vi "参数设置页.vi"() -> ()   [LabVIEW 2016, in "斯坦道总磷.lvlib"]
uses:
  <vilib>/Plasmionique/MB Master/MB_Master/MB_Master.lvclass
  <vilib>/ptbypt/NI_PtbyPt.lvlib
panel:
  in  "简易流程路径":path=path "data/流程.xml"
  out "数据刷新时间":string
  in  "通讯连接":bool
  out "MB table":enum32{"Serial", "TCP"}(tab)
  in  "请选择串口:":refnum<visa-resource-name>
  in  "IP":string="127.0.0.1"
  in  "PORT":string="1001"
  in  "通信方式选择":enum16{"串口", "TCP"}(ring)
  in  "盐度自动补偿：":bool
  out "盐度补偿值":dbl caption="盐度补偿值："
  in  "刷新":bool
  in  "测量模式":T1(ring)
  in  "参数下拉列表":u16(ring)
  in  "量程下拉列表":enum16{"低量程", "高量程"}(ring)
  in  "测试流程路径":path=path "data/流程.xml"
  in  "标样核查量程模式":enum16{"高量程", "低量程", "自动"}(ring) caption="标样核查量程模式："
  in  "加标回收量程模式":enum16{"高量程", "低量程", "自动"}(ring) caption="加标回收量程模式："
  in  "跨度核查量程模式":enum16{"高量程", "低量程", "自动"}(ring) caption="跨度核查量程模式："
  in  "零点核查量程模式":enum16{"高量程", "低量程", "自动"}(ring) caption="零点核查量程模式："
  in  "水样测试量程模式":enum16{"高量程", "低量程", "自动"}(ring) caption="水样测试量程模式："
  out "稀释度":dbl caption="稀释度："
  out "阈值（高->低）":dbl caption="阈值（高->低）："
  out "阈值（低->高）":dbl caption="阈值（低->高）："
  out "量程下限":dbl caption="量程下限："
  out "量程上限":dbl caption="量程上限："
  out "检出限":dbl caption="检出限："
  out "曲线截距":dbl caption="曲线截距：" format="%#.6f"
  out "曲线斜率":dbl caption="曲线斜率：" format="%#.6f"
  out "二次多项式系数":dbl caption="二次多项式系数：" format="%#.6f"
  out "消解时长":dbl caption="消解时长："
  out "消解温度":dbl caption="消解温度："
  out "测量精度":u16 caption="测量精度："
  in  "标样核查标液浓度":dbl caption="标样核查标液浓度："
  in  "跨度核查标液浓度":dbl caption="跨度核查标液浓度："
  in  "零点核查标液浓度":dbl caption="零点核查标液浓度："
  in  "跨度值":dbl caption="跨度值："
  # "ppt"
  # "mg/L"
  # "mg/L"
  # "mg/L"
  # "mg/L"
  # "mg/L"
  # "min"
  # "℃"
  # "mg/L"
  # "mg/L"
  # "mg/L"
  # "mg/L"
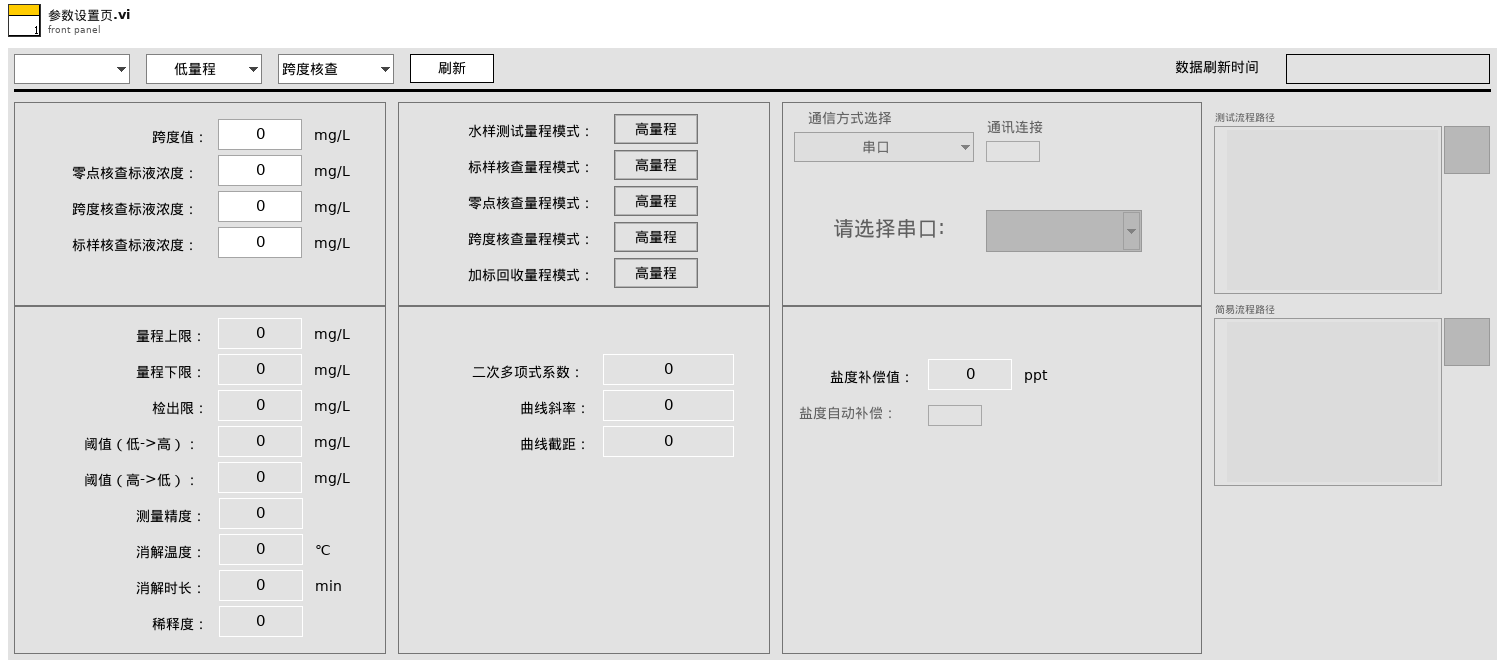
[diagram p1: front panel]
types:
  T1 = enum16{"跨度核查", "水样测量", "零点核查", "标样核查", "加标回收", "快捷测试", "空白校准", "标样校准"}
  T2 = typedef "LVStringsAndValuesArrayTypeDef_U16.ctl" = cluster{"String":string, "Value":u16}[]
  T3 = cluster{"系统时间":timestamp, "工作状态":u16, "测量模式":enum16{"待机", "连续模式", "周期模式", "定点模式", "受控模式", "手动模式"}, "告警代码":u16, "故障代码":u16, "日志代码":u16, "软件版本":u16, "F0":sgl, "F1":sgl, "F2":sgl, "F3":sgl, "T":sgl, "H":sgl, "id":u16, "flowid":u16, "量程":u16, "总磷控温温度1":sgl, "营养盐控温温度2":sgl, "ADC":sgl}
  T4 = enum8{"Enabled", "Disabled", "Disabled and Grayed Out"}
  T5 = cluster{"测量精度":u16, "检出限":dbl, "上限":dbl, "下限":dbl, "阈值（低->高）":dbl, "阈值（高->低）":dbl, "稀释度":dbl}
  T6 = cluster{"泵类型":u8, "进样速度":u32, "出样速度":u32, "泵阀量":u8, "光谱仪类型":u8, "光谱采样次数":u8, "氙灯次数":u8, "B":u16, "C":u16, "D":u16, "E":u16, "B_COD":u16, "C_COD":u16, "D_COD":u16, "E_COD":u16, "G":u16, "M":u16, "N":u16, "氨氮注射泵控温下限":sgl, "氨氮注射泵控温上限":sgl, "总氮注射泵控温下限":sgl, "总氮注射泵控温上限":sgl, "消解温度下限":sgl, "消解温度上限":sgl, "加热10s限值":sgl, "高温高压阀开阀温度":sgl, "总氮x公式0":u8, "总氮x公式1":sgl, "总氮x公式2":sgl, "总磷浊度稀释系数":sgl, "总磷浊度补偿权重1":sgl, "总磷浊度补偿权重2":sgl, "盐度系数":sgl, "氨氮补偿系数1":sgl, "氨氮补偿系数2":sgl}
  T7 = cluster{"水样测试量程模式":enum16{"高量程", "低量程", "自动"}, "零点核查量程模式":enum16{"高量程", "低量程", "自动"}, "跨度核查量程模式":enum16{"高量程", "低量程", "自动"}, "加标回收量程模式":enum16{"高量程", "低量程", "自动"}, "标样核查量程模式":enum16{"高量程", "低量程", "自动"}}
  T8 = cluster{"水样测试量程模式":u16, "零点核查量程模式":u16, "跨度核查量程模式":u16, "加标回收量程模式":u16, "标样核查量程模式":u16}
  T9 = cluster{"总磷跨度值":dbl, "总磷零点标准液浓度":dbl, "总磷跨度标准液浓度":dbl, "总磷标准液标准浓度":dbl, "总氮跨度值":dbl, "总氮零点标准液浓度":dbl, "总氮跨度标准液浓度":dbl, "总氮标准液标准浓度":dbl, "COD跨度值":dbl, "COD零点标准液浓度":dbl, "COD跨度标准液浓度":dbl, "COD标准液标准浓度":dbl, "氨氮跨度值":dbl, "氨氮零点标准液浓度":dbl, "氨氮跨度标准液浓度":dbl, "氨氮标准液标准浓度":dbl, "磷酸盐跨度值":dbl, "磷酸盐零点标准液浓度":dbl, "磷酸盐跨度标准液浓度":dbl, "磷酸盐标准液标准浓度":dbl, "硝氮跨度值":dbl, "硝氮零点标准液浓度":dbl, "硝氮跨度标准液浓度":dbl, "硝氮标准液标准浓度":dbl, "亚硝氮跨度值":dbl, "亚硝氮零点标准液浓度":dbl, "亚硝氮跨度标准液浓度":dbl, "亚硝氮标准液标准浓度":dbl, "硫化物跨度值":dbl, "硫化物零点标准液浓度":dbl, "硫化物跨度标准液浓度":dbl, "硫化物标准液标准浓度":dbl, "硅酸盐跨度值":dbl, "硅酸盐零点标准液浓度":dbl, "硅酸盐跨度标准液浓度":dbl, "硅酸盐标准液标准浓度":dbl}
  T10 = cluster{"水样测试量程模式":enum16{"H", "L", "AUTO"}, "空白核查量程模式":enum16{"H", "L", "AUTO"}, "跨度核查量程模式":enum16{"H", "L", "AUTO"}, "加标回收量程模式":enum16{"H", "L", "AUTO"}, "标样核查量程模式":enum16{"H", "L", "AUTO"}}
  T11 = cluster{"水样测试量程模式":u16, "空白核查量程模式":u16, "跨度核查量程模式":u16, "加标回收量程模式":u16, "标样核查量程模式":u16}
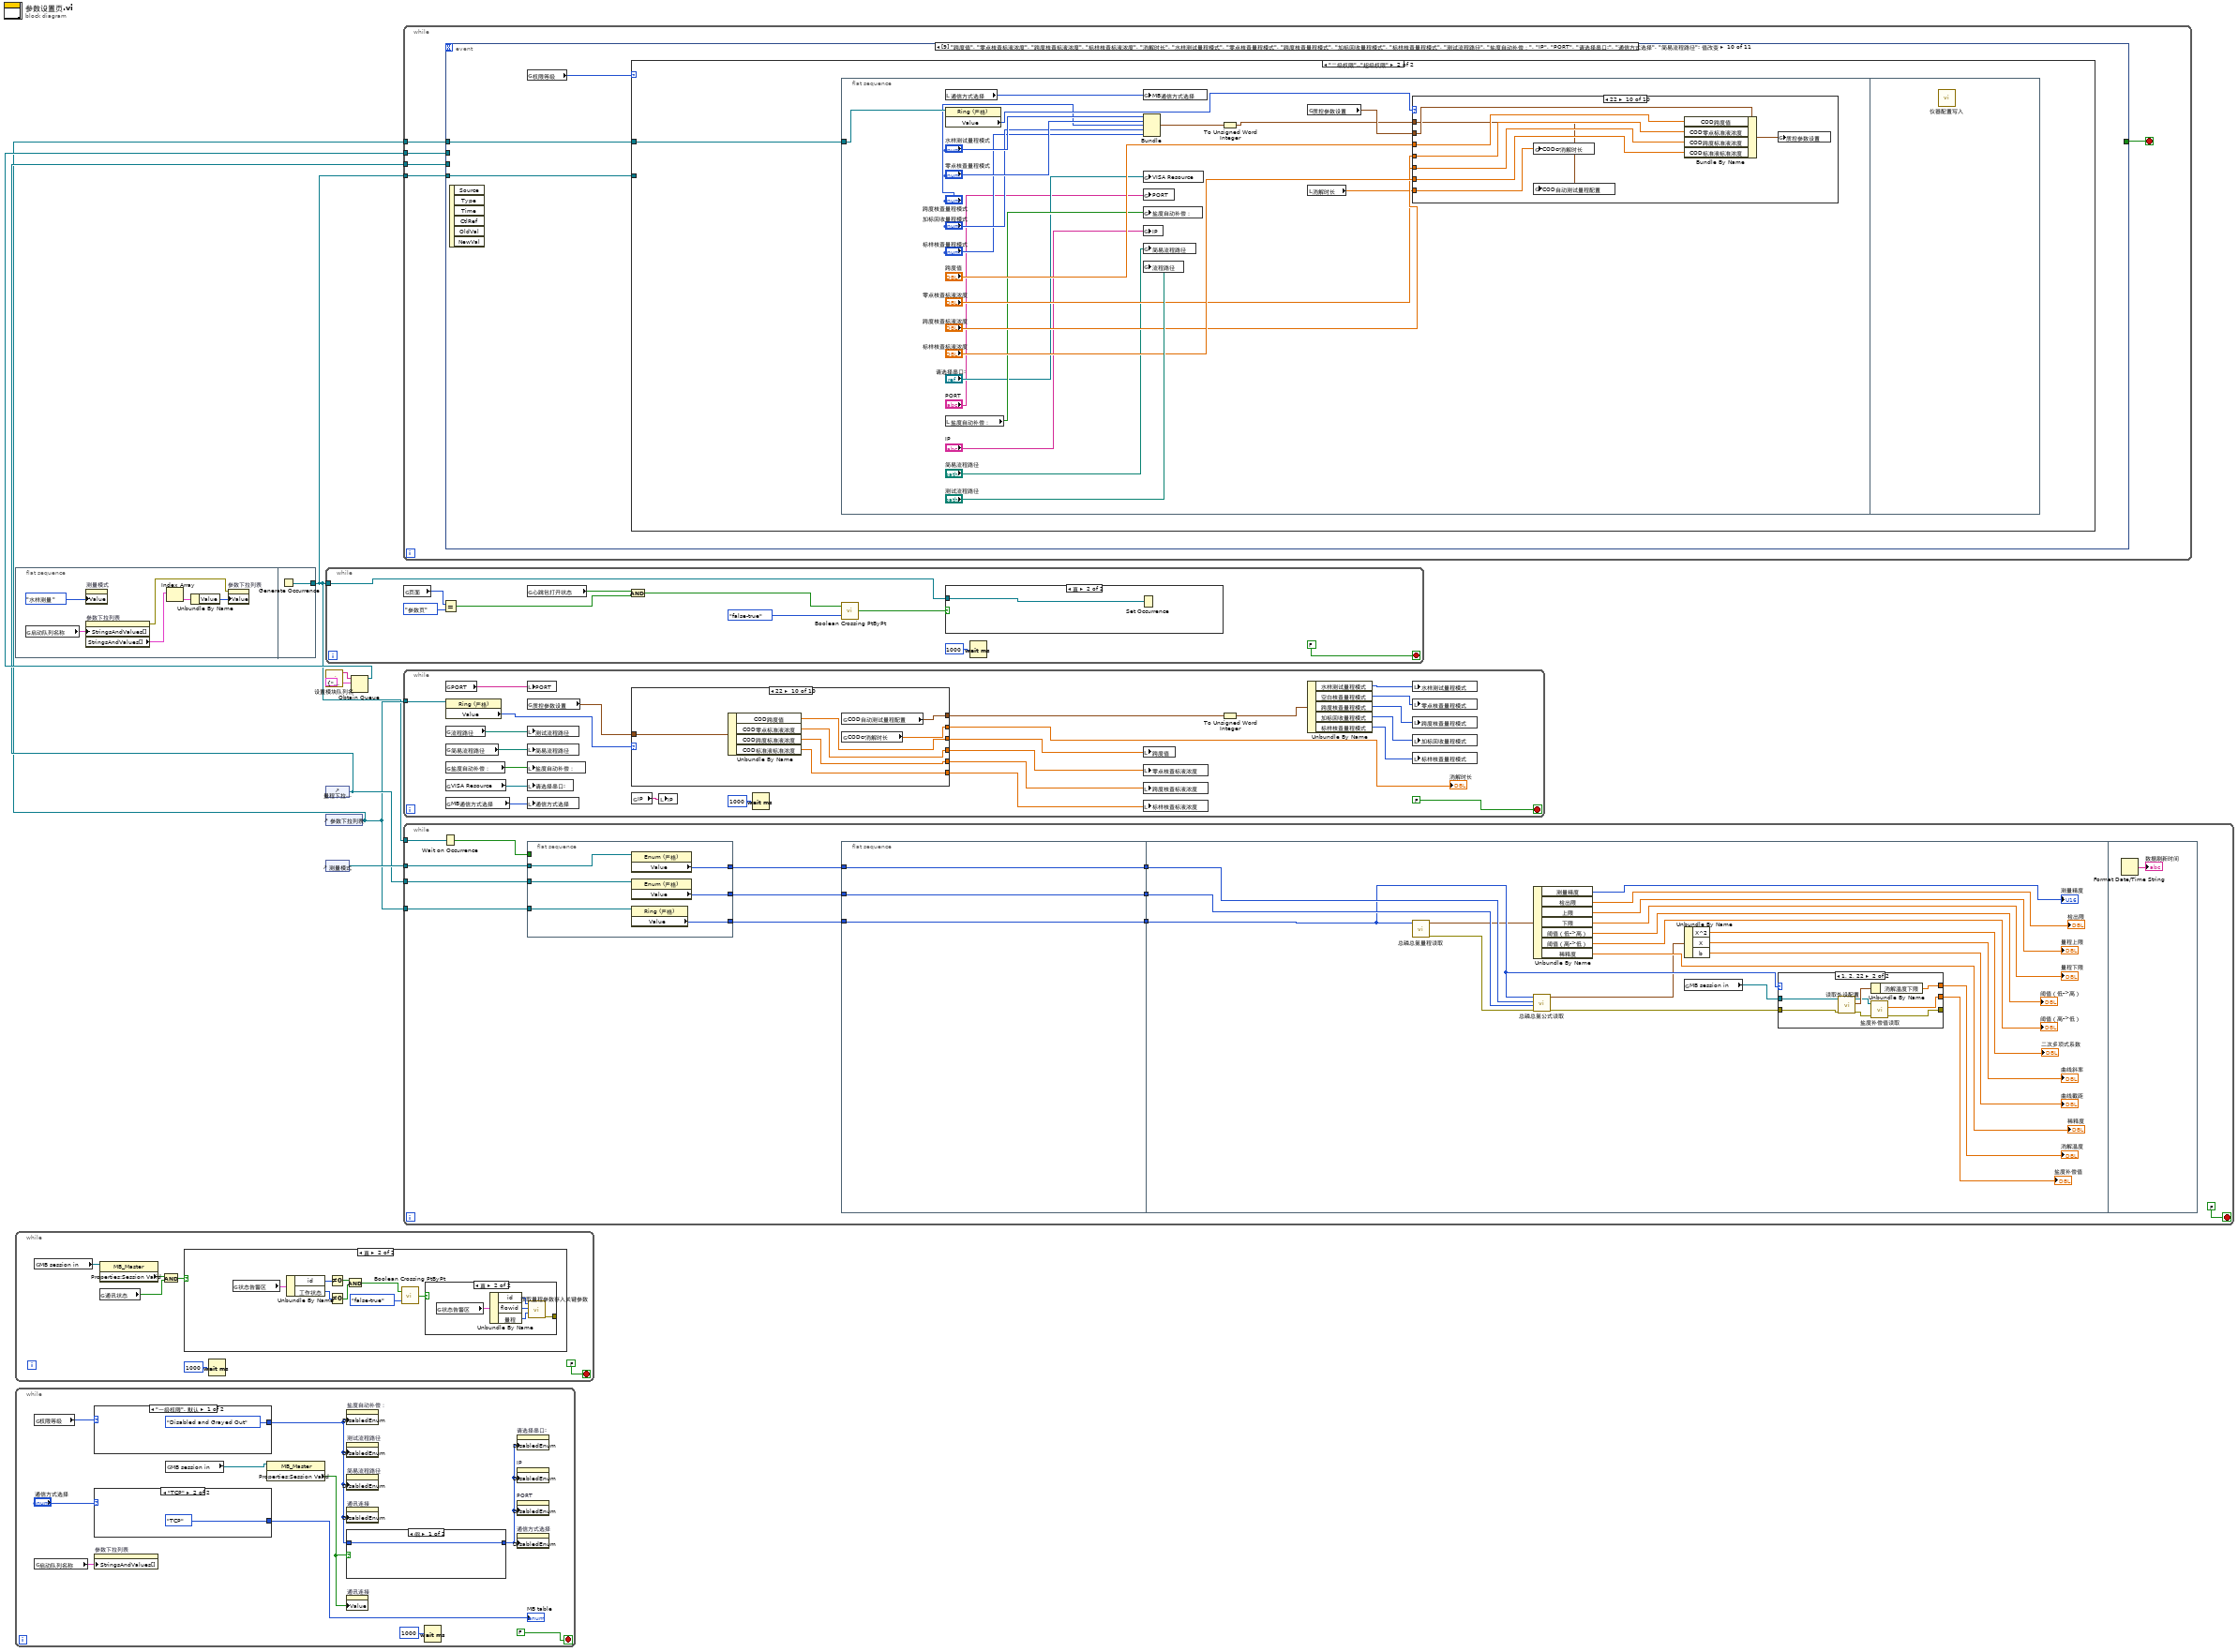
[diagram p0: block diagram]
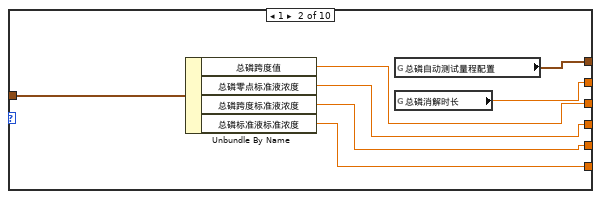
[diagram p6: hidden frame]
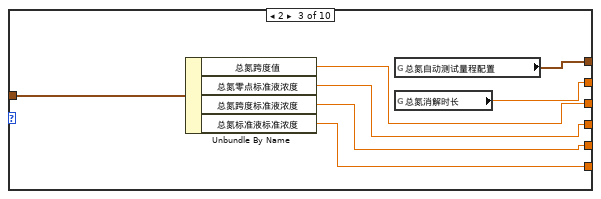
[diagram p7: hidden frame]
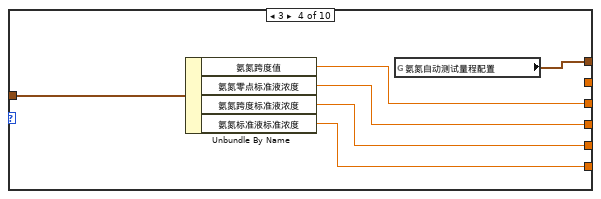
[diagram p8: hidden frame]
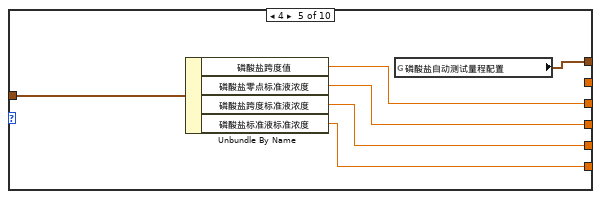
[diagram p9: hidden frame]
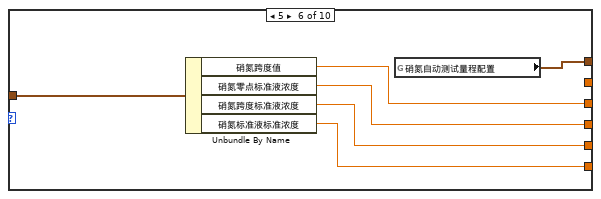
[diagram p10: hidden frame]
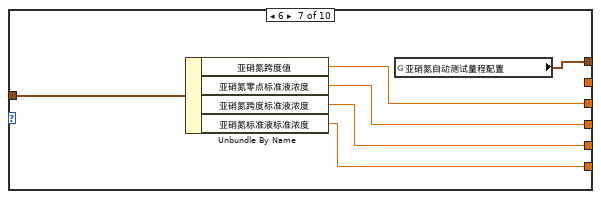
[diagram p11: hidden frame]
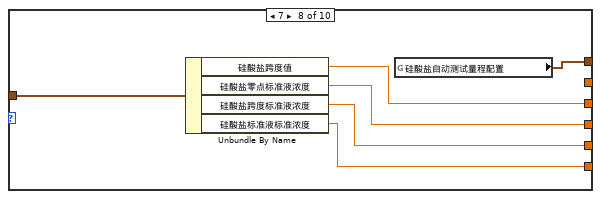
[diagram p12: hidden frame]
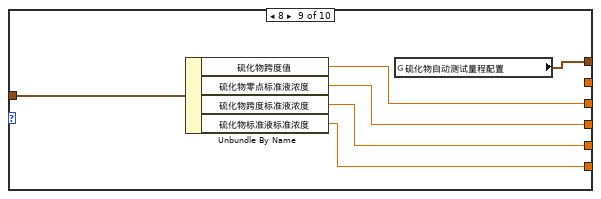
[diagram p13: hidden frame]
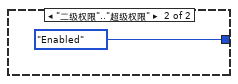
[diagram p14: hidden frame]
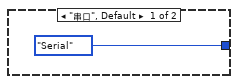
[diagram p15: hidden frame]
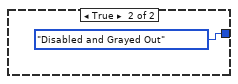
[diagram p16: hidden frame]
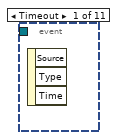
[diagram p17: hidden frame]
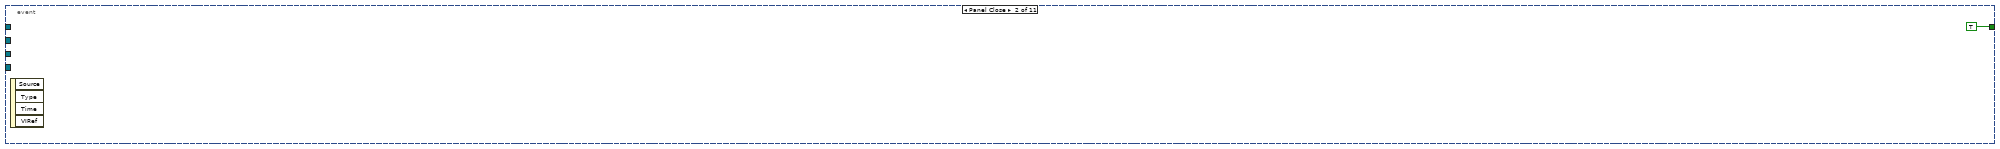
[diagram p18: hidden frame]
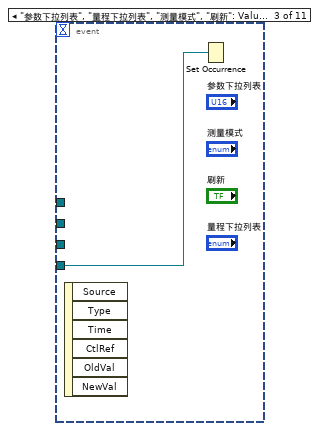
[diagram p19: hidden frame]
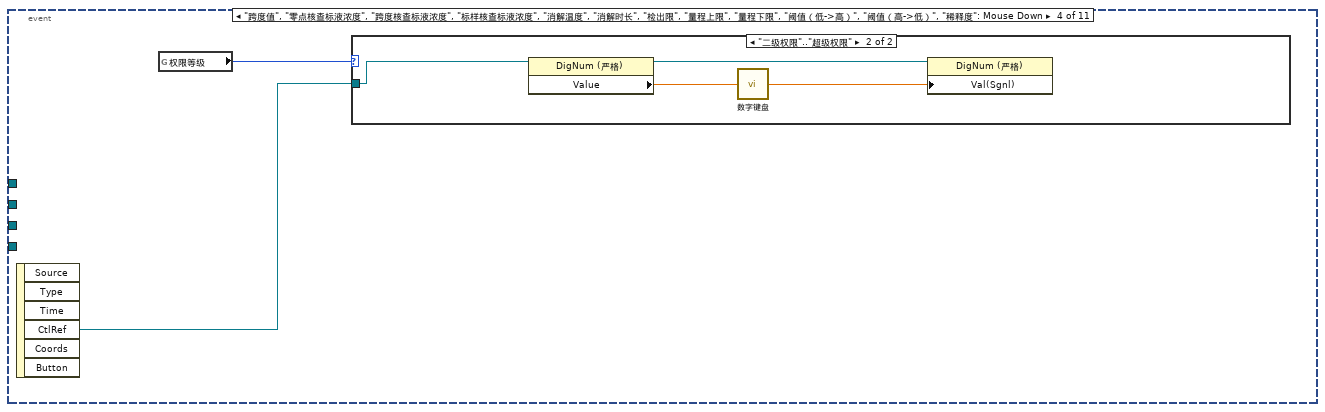
[diagram p20: hidden frame]
diagram:
  n1 = flat-sequence {
    tunnel: [w14] -> w1
    frame #0 {
      n2 = global read "model config var.vi" "启动队列名称"() -> (w9:cluster{"String":string, "Value":u16}[])
      n3 = property on="测量模式" class="Enum (严格)"("Value"=T1."水样测量" ("测量模式")) -> ()  [unwired: 2 in, 2 out]
      n4 = property on="参数下拉列表" class="Ring (严格)"("StringsAndValues[]"=w9) -> (error out=w12:errorcluster, "StringsAndValues[]"=w10:T2)  [unwired: 2 in, 1 out]
      n5 = Index Array(array=w10) -> (element=w11:cluster{"String":string, "Value":u16})  [unwired: 1 in]
      n6 = Unbundle By Name(w11) -> ("Value"=w13:u16)
      n7 = property on="参数下拉列表" class="Ring (严格)"(error in=w12, "Value"=w13) -> ()  [unwired: 1 in, 2 out]
    }
    frame #1 {
      n8 = Generate Occurrence() -> (w14:refnum<k4>)
    }
  }
  n9 = while {
    stop <- FALSE stop-if-true
    n10 = global read "VAR总磷总氮全局变量.vi" "MB session in"() -> (w17:refnum<class "MB_Master.lvclass">)
    n11 = property class="MB_Master"(reference=w17) -> ("Properties:Session Valid"=w15:bool)  [unwired: 1 in, 2 out]
    n12 = global read "VAR总磷总氮全局变量.vi" "通讯状态"() -> (w19:bool)
    n13 = And(x=w15, y=w19) -> (x .and. y?=w16:bool)
    n14 = case shown="真" w16 {
      frame False {
      }
      frame True {
        n15 = global read "VAR总磷总氮全局变量.vi" "状态告警区"() -> (w28:T3)
        n16 = Unbundle By Name(w28) -> ("id"=w22:u16, "工作状态"=w27:u16)
        n17 = Not Equal To 0?(x=w22) -> (x != 0?=w23:bool)
        n18 = Not Equal To 0?(x=w27) -> (x != 0?=w24:bool)
        n19 = And(x=w23, y=w24) -> (x .and. y?=w25:bool)
        n20 = call <vilib>:"Boolean Crossing PtByPt.vi"("direction"=enum16{"either", "false-true", "true-false"}."false-true", "input"=w25) -> ("crossing"=w21:bool)  [unwired: 1 in]
        n21 = case shown="真" w21 {
          tunnel: [_ w33] -> _
          frame False {
          }
          frame True {
            n22 = global read "VAR总磷总氮全局变量.vi" "状态告警区"() -> (w32:T3)
            n23 = Unbundle By Name(w32) -> ("id"=w31:u16, "flowid"=w30:u16, "量程"=w29:u16)
            n24 = call "获取量程参数存入关键参数.vi"("量程"=w29, "flowid"=w30, "id"=w31) -> ("error out"=w33:errorcluster)  [unwired: 8 in]
          }
        }
      }
    }
    n25 = Wait (ms)(milliseconds to wait=u32 1000 ("等待时间（毫秒）")) -> ()  [unwired: 1 out]
  }
  n26 = while {
    stop <- FALSE stop-if-true
    n27 = global read "VAR总磷总氮全局变量.vi" "权限等级"() -> (w36:enum16{"一级权限", "二级权限", "三级权限", "超级权限"})
    n28 = global read "model config var.vi" "启动队列名称"() -> (w34:cluster{"String":string, "Value":u16}[])
    n29 = case shown="\"一级权限\", 默认" w36 {
      tunnel: [T4."Disabled and Grayed Out" ("禁用") T4."Enabled" ("禁用")] -> w35
      frame "一级权限", Default {
      }
      frame "二级权限".."超级权限" {
      }
    }
    n30 = case shown="\"TCP\"" "通信方式选择" {
      tunnel: [enum32{"Serial", "TCP"}."Serial" ("MB table") enum32{"Serial", "TCP"}."TCP" ("MB table")] -> w38
      frame "串口", Default {
      }
      frame "TCP" {
      }
    }
    "MB table" <- w38
    n31 = property on="参数下拉列表" class="Ring (严格)"("StringsAndValues[]"=w34) -> ()  [unwired: 2 in, 2 out]
    n32 = global read "VAR总磷总氮全局变量.vi" "MB session in"() -> (w42:refnum<class "MB_Master.lvclass">)
    n33 = property class="MB_Master"(reference=w42) -> ("Properties:Session Valid"=w40:bool)  [unwired: 1 in, 2 out]
    n34 = property on="盐度自动补偿：" class="Bool (严格)"("DisabledEnum"=w35) -> ()  [unwired: 2 in, 2 out]
    n35 = property on="测试流程路径" class="Path"("DisabledEnum"=w35) -> ()  [unwired: 2 in, 2 out]
    n36 = property on="简易流程路径" class="Path"("DisabledEnum"=w35) -> ()  [unwired: 2 in, 2 out]
    n37 = property on="通讯连接" class="Bool (严格)"("DisabledEnum"=w35) -> ()  [unwired: 2 in, 2 out]
    n38 = case shown="假" w40 {
      tunnel: [w48 T4."Disabled and Grayed Out" ("禁用")] -> w39
      tunnel: w35 -> [w48 _]
      frame False {
      }
      frame True {
      }
    }
    n39 = property on="通讯连接" class="Bool (严格)"("Value"=w40) -> ()  [unwired: 2 in, 2 out]
    n40 = Wait (ms)(milliseconds to wait=u32 1000 ("等待时间（毫秒）")) -> ()  [unwired: 1 out]
    n41 = property on="请选择串口:" class="VISAName"("DisabledEnum"=w39) -> ()  [unwired: 2 in, 2 out]
    n42 = property on="IP" class="Str"("DisabledEnum"=w39) -> ()  [unwired: 2 in, 2 out]
    n43 = property on="PORT" class="Str"("DisabledEnum"=w39) -> ()  [unwired: 2 in, 2 out]
    n44 = property on="通信方式选择" class="Enum (严格)"("DisabledEnum"=w39) -> ()  [unwired: 2 in, 2 out]
  }
  n45 = while {
    tunnel: w1 -> [w56]
    stop <- FALSE stop-if-true
    n46 = global read "VAR总磷总氮全局变量.vi" "页面"() -> (w58:enum16{"主页", "参数页", "校准页"})
    n47 = Equal?(x=w58, y=enum16{"主页", "参数页", "校准页"}."参数页" ("页面")) -> (x = y?=w57:bool)
    n48 = global read "VAR总磷总氮全局变量.vi" "心跳包打开状态"() -> (w52:bool)
    n49 = And(x=w52, y=w57) -> (x .and. y?=w53:bool)
    n50 = call <vilib>:"Boolean Crossing PtByPt.vi"("direction"=enum16{"either", "false-true", "true-false"}."false-true", "input"=w53) -> ("crossing"=w51:bool)  [unwired: 1 in]
    n51 = case shown="真" w51 {
      tunnel: w56 -> [_ w60]
      frame False {
      }
      frame True {
        n52 = Set Occurrence(w60) -> ()
      }
    }
    n53 = Wait (ms)(milliseconds to wait=u32 1000 ("等待时间（毫秒）")) -> ()  [unwired: 1 out]
  }
  n54 = call "设置模块队列名.vi"() -> ("Msg"=w6:string)  [unwired: 5 in]
  n55 = control-ref of="量程下拉列表"() -> (w3:refnum<vi>)
  n56 = control-ref of="参数下拉列表"() -> (w2:refnum<vi>)
  n57 = control-ref of="测量模式"() -> (w4:refnum<vi>)
  n58 = Obtain Queue(name (unnamed)=w6, element data type=cluster{"命令":string, "data":variant} {"命令"="", "data"=variant}) -> (queue out=w5:refnum<queue>)  [unwired: 3 in, 2 out]
  n59 = while {
    tunnel: w1 -> [w64]
    tunnel: w2 -> [w63]
    tunnel: w5 -> [w62]
    tunnel: w3 -> [w61]
    stop <- w65 stop-if-true
    n60 = event shown="[9] \"跨度值\", \"零点核查标液浓度\", \"跨度核查标液浓度\", \"标样核查标液浓度\", \"消解时长\", \"水样测试量程模式\", \"零点核查量程模式\", \"跨度核查量程模式\", \"加标回收量程模式\", \"标样核查量程模式\", \"测试流程路径\", \"盐度自动补偿：\", \"IP\", \"PORT\", \"请选择串口:\", \"通信方式选择\", \"简易流程路径\": 值改变" {
      selector: _ -> [_ _ _ _ _ _ _ _ _ _ _]
      dyn-events: _ -> [_ _ _ _ _ _ _ _ _ _ _]
      timeout: _ -> [_ _ _ _ _ _ _ _ _ _ _]
      tunnel: [_ TRUE _ _ _ _ _ _ _ _ _] -> w65
      tunnel: w64 -> [_ _ w67 _ _ _ _ _ _ w114 _]
      tunnel: w63 -> [_ _ _ _ w86 _ _ _ _ w116 _]
      tunnel: w62 -> [_ _ _ _ _ _ _ _ _ _ w208]
      tunnel: w61 -> [_ _ _ _ _ _ _ _ _ _ _]
      event Timeout {
        n61 = event-data() -> ()  [unwired: 1 in, 3 out]
      }
      event Panel Close {
        n62 = event-data() -> ()  [unwired: 1 in, 4 out]
      }
      event "参数下拉列表", "量程下拉列表", "测量模式", "刷新": Value Change {
        n63 = event-data() -> ()  [unwired: 1 in, 6 out]
        n64 = Set Occurrence(w67) -> ()
      }
      event "跨度值", "零点核查标液浓度", "跨度核查标液浓度", "标样核查标液浓度", "消解温度", "消解时长", "检出限", "量程上限", "量程下限", "阈值（低->高）", "阈值（高->低）", "稀释度": Mouse Down {
        n65 = event-data() -> ("CtlRef"=w69:refnum<vi>)  [unwired: 1 in, 5 out]
        n66 = global read "VAR总磷总氮全局变量.vi" "权限等级"() -> (w68:enum16{"一级权限", "二级权限", "三级权限", "超级权限"})
        n67 = case shown="\"二级权限\"..\"超级权限\"" w68 {
          tunnel: w69 -> [_ w73]
          frame "一级权限", Default {
          }
          frame "二级权限".."超级权限" {
            n68 = property class="DigNum (严格)"(reference=w73) -> (reference out=w71:refnum<vi>, "Value"=w72:dbl)  [unwired: 1 in, 1 out]
            n69 = call "数字键盘.vi"("OldNumber"=w72) -> ("NewNumber"=w70:dbl)
            n70 = property class="DigNum (严格)"(reference=w71, "Val(Sgnl)"=w70) -> ()  [unwired: 1 in, 2 out]
          }
        }
      }
      event "测量精度", "检出限", "量程上限", "量程下限", "阈值（低->高）", "阈值（高->低）", "稀释度": Value Change {
        n71 = event-data() -> ()  [unwired: 1 in, 6 out]
        n72 = local read "测量精度"() -> (w76:u16)
        n73 = local read "检出限"() -> (w80:dbl)
        n74 = local read "量程上限"() -> (w82:dbl)
        n75 = local read "量程下限"() -> (w81:dbl)
        n76 = local read "阈值（低->高）"() -> (w79:dbl)
        n77 = local read "阈值（高->低）"() -> (w78:dbl)
        n78 = local read "稀释度"() -> (w77:dbl)
        n79 = property class="Ring (严格)"(reference=w86) -> ("Value"=w85:u16)  [unwired: 1 in, 2 out]
        n80 = Bundle By Name(cluster=T5 {"测量精度"=0, "检出限"=0.0, "上限"=0.0, "下限"=0.0, "阈值（低->高）"=0.0, "阈值（高->低）"=0.0, "稀释度"=0.0} ("量程参数写入"), "测量精度"=w76, "检出限"=w80, "上限"=w82, "下限"=w81, "阈值（低->高）"=w79, "阈值（高->低）"=w78, "稀释度"=w77) -> (w83:T5)
        n81 = call "总磷总氮量程写入.vi"("量程参数写入"=w83, "测量参数"=w85) -> ("error out"=w74:errorcluster)  [unwired: 8 in]
        n82 = case shown="错误" w74 {
          tunnel: ["写入成功" "写入失败"] -> w75
          frame No Error {
          }
          frame Error {
          }
        }
        n83 = One Button Dialog(message=w75) -> ()  [unwired: 1 in, 1 out]
      }
      event "消解温度": Value Change {
        n84 = event-data() -> ("NewVal"=w91:dbl)  [unwired: 1 in, 5 out]
        n85 = global read "VAR总磷总氮全局变量.vi" "MB session in"() -> (w92:refnum<class "MB_Master.lvclass">)
        n86 = call "读取外设配置.vi"("MB session in"=w92) -> ("error out"=w95:errorcluster, "外设配置"=w94:T6)  [unwired: 8 in, 1 out]
        n87 = Bundle By Name(cluster=w94, "消解温度下限"=w91) -> (w93:T6)
        n88 = call "写入外设配置.vi"("error in (no error)"=w95, "外设配置"=w93, "MB session in"=w92) -> ("error out"=w90:errorcluster)  [unwired: 7 in, 1 out]
        n89 = case shown="错误" w90 {
          tunnel: ["写入成功" "写入失败"] -> w89
          frame No Error {
          }
          frame Error {
          }
        }
        n90 = One Button Dialog(message=w89) -> ()  [unwired: 1 in, 1 out]
      }
      event "测量精度": Mouse Down {
        n91 = event-data() -> ("CtlRef"=w99:refnum<vi>)  [unwired: 1 in, 7 out]
        n92 = global read "VAR总磷总氮全局变量.vi" "权限等级"() -> (w98:enum16{"一级权限", "二级权限", "三级权限", "超级权限"})
        n93 = case shown="\"二级权限\"..\"超级权限\"" w98 {
          tunnel: w99 -> [_ w103]
          frame "一级权限", Default {
          }
          frame "二级权限".."超级权限" {
            n94 = property class="DigNum (严格)"(reference=w103) -> (reference out=w101:refnum<vi>, "Value"=w102:u16)  [unwired: 1 in, 1 out]
            n95 = call "数字键盘.vi"("OldNumber"=w102) -> ("NewNumber"=w100:dbl)
            n96 = property class="DigNum (严格)"(reference=w101, "Val(Sgnl)"=w100) -> ()  [unwired: 1 in, 2 out]
          }
        }
      }
      event "盐度补偿值": Mouse Down {
        n97 = event-data() -> ("CtlRef"=w105:refnum<vi>)  [unwired: 1 in, 3 out]
        n98 = global read "VAR总磷总氮全局变量.vi" "权限等级"() -> (w104:enum16{"一级权限", "二级权限", "三级权限", "超级权限"})
        n99 = case shown="\"二级权限\"..\"超级权限\"" w104 {
          tunnel: w105 -> [_ w107]
          frame "一级权限", Default {
          }
          frame "二级权限".."超级权限" {
            n100 = case shown="假" "盐度自动补偿：" {
              tunnel: w107 -> [w111 _]
              frame False {
                n101 = property class="DigNum (严格)"(reference=w111) -> (reference out=w109:refnum<vi>, "Value"=w110:dbl)  [unwired: 1 in, 1 out]
                n102 = call "数字键盘.vi"("OldNumber"=w110) -> ("NewNumber"=w108:dbl)
                n103 = property class="DigNum (严格)"(reference=w109, "Val(Sgnl)"=w108) -> ()  [unwired: 1 in, 2 out]
              }
              frame True {
              }
            }
          }
        }
      }
      event "盐度补偿值": Value Change {
        n104 = event-data() -> ("NewVal"=w112:dbl)  [unwired: 1 in, 5 out]
        n105 = global read "VAR总磷总氮全局变量.vi" "MB session in"() -> (w113:refnum<class "MB_Master.lvclass">)
        n106 = call "盐度补偿值写入.vi"("盐度补偿值"=w112, "MB session in"=w113) -> ()  [unwired: 8 in, 2 out]
      }
      event "跨度值", "零点核查标液浓度", "跨度核查标液浓度", "标样核查标液浓度", "消解时长", "水样测试量程模式", "零点核查量程模式", "跨度核查量程模式", "加标回收量程模式", "标样核查量程模式", "测试流程路径", "盐度自动补偿：", "IP", "PORT", "请选择串口:", "通信方式选择", "简易流程路径": Value Change {
        n107 = event-data() -> ()  [unwired: 1 in, 6 out]
        n108 = global read "VAR总磷总氮全局变量.vi" "权限等级"() -> (w115:enum16{"一级权限", "二级权限", "三级权限", "超级权限"})
        n109 = case shown="\"二级权限\"..\"超级权限\"" w115 {
          tunnel: w116 -> [_ w118]
          tunnel: w114 -> [w117 _]
          frame "一级权限", Default {
            n110 = Set Occurrence(w117) -> ()
          }
          frame "二级权限".."超级权限" {
            n111 = flat-sequence {
              tunnel: w118 -> [w139]
              frame #0 {
                n112 = local read "通信方式选择"() -> (w121:enum16{"串口", "TCP"})
                n113 = property class="Ring (严格)"(reference=w139) -> ("Value"=w138:u16)  [unwired: 1 in, 2 out]
                n114 = local read "盐度自动补偿："() -> (w125:bool)
                n115 = global write "总磷总氮断电保存全局变量.vi" "MB通信方式选择"(w121) -> ()
                n116 = Bundle("水样测试量程模式"="水样测试量程模式", "零点核查量程模式"="零点核查量程模式", "跨度核查量程模式"="跨度核查量程模式", "加标回收量程模式"="加标回收量程模式", "标样核查量程模式"="标样核查量程模式") -> (w127:T7)  [unwired: 1 in]
                n117 = global write "总磷总氮断电保存全局变量.vi" "VISA Resource"("请选择串口:") -> ()
                n118 = global write "总磷总氮断电保存全局变量.vi" "PORT"("PORT") -> ()
                n119 = global write "总磷总氮断电保存全局变量.vi" "盐度自动补偿："(w125) -> ()
                n120 = global write "总磷总氮断电保存全局变量.vi" "IP"("IP") -> ()
                n121 = global write "总磷总氮断电保存全局变量.vi" "简易流程路径"("简易流程路径") -> ()
                n122 = global write "总磷总氮断电保存全局变量.vi" "流程路径"("测试流程路径") -> ()
                n123 = To Unsigned Word Integer(number=w127) -> (unsigned 16bit integer=w126:T8)
                n124 = global read "总磷总氮断电保存全局变量.vi" "质控参数设置"() -> (w133:T9)
                n125 = local read "消解时长"() -> (w120:dbl)
                n126 = case shown="22" w138 {
                  tunnel: "跨度值" -> [_ w146 w154 w161 w168 w175 w182 w189 w196 w204]
                  tunnel: "标样核查标液浓度" -> [_ w143 w151 w158 w165 w172 w179 w186 w193 w201]
                  tunnel: "跨度核查标液浓度" -> [_ w144 w152 w159 w166 w173 w180 w187 w194 w202]
                  tunnel: "零点核查标液浓度" -> [_ w145 w153 w160 w167 w174 w181 w188 w195 w203]
                  tunnel: w133 -> [_ w148 w156 w163 w170 w177 w184 w191 w198 w206]
                  tunnel: w126 -> [_ w142 w150 w157 w164 w171 w178 w185 w192 w199]
                  tunnel: w120 -> [_ w141 w149 _ _ _ _ _ _ w200]
                  frame 0, Default {
                  }
                  frame 1 {
                    n127 = global write "总磷总氮断电保存全局变量.vi" "总磷自动测试量程配置"(w142) -> ()
                    n128 = global write "总磷总氮断电保存全局变量.vi" "总磷消解时长"(w141) -> ()
                    n129 = Bundle By Name(cluster=w148, "总磷跨度值"=w146, "总磷零点标准液浓度"=w145, "总磷跨度标准液浓度"=w144, "总磷标准液标准浓度"=w143) -> (w147:T9)
                    n130 = global write "总磷总氮断电保存全局变量.vi" "质控参数设置"(w147) -> ()
                  }
                  frame 2 {
                    n131 = global write "总磷总氮断电保存全局变量.vi" "总氮自动测试量程配置"(w150) -> ()
                    n132 = global write "总磷总氮断电保存全局变量.vi" "总氮消解时长"(w149) -> ()
                    n133 = Bundle By Name(cluster=w156, "总氮跨度值"=w154, "总氮零点标准液浓度"=w153, "总氮跨度标准液浓度"=w152, "总氮标准液标准浓度"=w151) -> (w155:T9)
                    n134 = global write "总磷总氮断电保存全局变量.vi" "质控参数设置"(w155) -> ()
                  }
                  frame 3 {
                    n135 = global write "总磷总氮断电保存全局变量.vi" "氨氮自动测试量程配置"(w157) -> ()
                    n136 = Bundle By Name(cluster=w163, "氨氮跨度值"=w161, "氨氮零点标准液浓度"=w160, "氨氮跨度标准液浓度"=w159, "氨氮标准液标准浓度"=w158) -> (w162:T9)
                    n137 = global write "总磷总氮断电保存全局变量.vi" "质控参数设置"(w162) -> ()
                  }
                  frame 4 {
                    n138 = global write "总磷总氮断电保存全局变量.vi" "磷酸盐自动测试量程配置"(w164) -> ()
                    n139 = Bundle By Name(cluster=w170, "磷酸盐跨度值"=w168, "磷酸盐零点标准液浓度"=w167, "磷酸盐跨度标准液浓度"=w166, "磷酸盐标准液标准浓度"=w165) -> (w169:T9)
                    n140 = global write "总磷总氮断电保存全局变量.vi" "质控参数设置"(w169) -> ()
                  }
                  frame 5 {
                    n141 = global write "总磷总氮断电保存全局变量.vi" "硝氮自动测试量程配置"(w171) -> ()
                    n142 = Bundle By Name(cluster=w177, "硝氮跨度值"=w175, "硝氮零点标准液浓度"=w174, "硝氮跨度标准液浓度"=w173, "硝氮标准液标准浓度"=w172) -> (w176:T9)
                    n143 = global write "总磷总氮断电保存全局变量.vi" "质控参数设置"(w176) -> ()
                  }
                  frame 6 {
                    n144 = global write "总磷总氮断电保存全局变量.vi" "亚硝氮自动测试量程配置"(w178) -> ()
                    n145 = Bundle By Name(cluster=w184, "亚硝氮跨度值"=w182, "亚硝氮零点标准液浓度"=w181, "亚硝氮跨度标准液浓度"=w180, "亚硝氮标准液标准浓度"=w179) -> (w183:T9)
                    n146 = global write "总磷总氮断电保存全局变量.vi" "质控参数设置"(w183) -> ()
                  }
                  frame 7 {
                    n147 = global write "总磷总氮断电保存全局变量.vi" "硅酸盐自动测试量程配置"(w185) -> ()
                    n148 = Bundle By Name(cluster=w191, "硅酸盐跨度值"=w189, "硅酸盐零点标准液浓度"=w188, "硅酸盐跨度标准液浓度"=w187, "硅酸盐标准液标准浓度"=w186) -> (w190:T9)
                    n149 = global write "总磷总氮断电保存全局变量.vi" "质控参数设置"(w190) -> ()
                  }
                  frame 8 {
                    n150 = global write "总磷总氮断电保存全局变量.vi" "硫化物自动测试量程配置"(w192) -> ()
                    n151 = Bundle By Name(cluster=w198, "硫化物跨度值"=w196, "硫化物零点标准液浓度"=w195, "硫化物跨度标准液浓度"=w194, "硫化物标准液标准浓度"=w193) -> (w197:T9)
                    n152 = global write "总磷总氮断电保存全局变量.vi" "质控参数设置"(w197) -> ()
                  }
                  frame 22 {
                    n153 = global write "总磷总氮断电保存全局变量.vi" "CODcr消解时长"(w200) -> ()
                    n154 = global write "总磷总氮断电保存全局变量.vi" "COD自动测试量程配置"(w199) -> ()
                    n155 = Bundle By Name(cluster=w206, "COD跨度值"=w204, "COD零点标准液浓度"=w203, "COD跨度标准液浓度"=w202, "COD标准液标准浓度"=w201) -> (w205:T9)
                    n156 = global write "总磷总氮断电保存全局变量.vi" "质控参数设置"(w205) -> ()
                  }
                }
              }
              frame #1 {
                n157 = call "仪器配置写入.vi"() -> ()  [unwired: 11 in, 1 out]
              }
            }
          }
        }
      }
      event "通讯连接": Value Change {
        n158 = event-data() -> ("NewVal"=w207:bool)  [unwired: 1 in, 5 out]
        n159 = Flush Queue(queue=w208) -> (queue out=w209:refnum<queue>)  [unwired: 1 in, 2 out]
        n160 = case shown="假" w207 {
          tunnel: w209 -> [w210 w212]
          frame False {
            n161 = Enqueue Element At Opposite End(queue=w210, element=cluster{"命令":string, "data":variant} {"命令"="停用模块", "data"=variant} ("元素")) -> ()  [unwired: 2 in, 3 out]
          }
          frame True {
            n162 = Enqueue Element At Opposite End(queue=w212, element=cluster{"命令":string, "data":variant} {"命令"="启用模块", "data"=variant} ("元素")) -> ()  [unwired: 2 in, 3 out]
          }
        }
      }
    }
  }
  n163 = while {
    tunnel: w2 -> [w216]
    stop <- FALSE stop-if-true
    n164 = global read "总磷总氮断电保存全局变量.vi" "PORT"() -> (w234:string)
    n165 = property class="Ring (严格)"(reference=w216) -> ("Value"=w215:u16)  [unwired: 1 in, 2 out]
    n166 = global read "总磷总氮断电保存全局变量.vi" "流程路径"() -> (w232:path)
    n167 = global read "总磷总氮断电保存全局变量.vi" "简易流程路径"() -> (w214:path)
    n168 = global read "总磷总氮断电保存全局变量.vi" "盐度自动补偿："() -> (w231:bool)
    n169 = global read "总磷总氮断电保存全局变量.vi" "VISA Resource"() -> (w235:refnum<visa-resource-name>)
    n170 = global read "总磷总氮断电保存全局变量.vi" "MB通信方式选择"() -> (w230:enum16{"串口", "TCP"})
    n171 = local write "PORT"(w234) -> ()
    n172 = global read "总磷总氮断电保存全局变量.vi" "质控参数设置"() -> (w225:T9)
    n173 = local write "测试流程路径"(w232) -> ()
    n174 = local write "简易流程路径"(w214) -> ()
    n175 = local write "盐度自动补偿："(w231) -> ()
    n176 = local write "请选择串口:"(w235) -> ()
    n177 = local write "通信方式选择"(w230) -> ()
    n178 = case shown="22" w215 {
      tunnel: [_ w244 w251 w257 w263 w269 w275 w281 w287 w294] -> w223
      tunnel: [_ w243 w250 _ _ _ _ _ _ w293] -> w224
      tunnel: w225 -> [_ w242 w249 w256 w262 w268 w274 w280 w286 w292]
      tunnel: [_ w241 w248 w255 w261 w267 w273 w279 w285 w291] -> w226
      tunnel: [_ w240 w247 w254 w260 w266 w272 w278 w284 w290] -> w227
      tunnel: [_ w239 w246 w253 w259 w265 w271 w277 w283 w289] -> w228
      tunnel: [_ w238 w245 w252 w258 w264 w270 w276 w282 w288] -> w229
      frame Default {
      }
      frame 1 {
        n179 = Unbundle By Name(w242) -> ("总磷跨度值"=w241:dbl, "总磷零点标准液浓度"=w240:dbl, "总磷跨度标准液浓度"=w239:dbl, "总磷标准液标准浓度"=w238:dbl)
        n180 = global read "总磷总氮断电保存全局变量.vi" "总磷自动测试量程配置"() -> (w244:T10)
        n181 = global read "总磷总氮断电保存全局变量.vi" "总磷消解时长"() -> (w243:dbl)
      }
      frame 2 {
        n182 = Unbundle By Name(w249) -> ("总氮跨度值"=w248:dbl, "总氮零点标准液浓度"=w247:dbl, "总氮跨度标准液浓度"=w246:dbl, "总氮标准液标准浓度"=w245:dbl)
        n183 = global read "总磷总氮断电保存全局变量.vi" "总氮自动测试量程配置"() -> (w251:T10)
        n184 = global read "总磷总氮断电保存全局变量.vi" "总氮消解时长"() -> (w250:dbl)
      }
      frame 3 {
        n185 = Unbundle By Name(w256) -> ("氨氮跨度值"=w255:dbl, "氨氮零点标准液浓度"=w254:dbl, "氨氮跨度标准液浓度"=w253:dbl, "氨氮标准液标准浓度"=w252:dbl)
        n186 = global read "总磷总氮断电保存全局变量.vi" "氨氮自动测试量程配置"() -> (w257:T10)
      }
      frame 4 {
        n187 = Unbundle By Name(w262) -> ("磷酸盐跨度值"=w261:dbl, "磷酸盐零点标准液浓度"=w260:dbl, "磷酸盐跨度标准液浓度"=w259:dbl, "磷酸盐标准液标准浓度"=w258:dbl)
        n188 = global read "总磷总氮断电保存全局变量.vi" "磷酸盐自动测试量程配置"() -> (w263:T10)
      }
      frame 5 {
        n189 = Unbundle By Name(w268) -> ("硝氮跨度值"=w267:dbl, "硝氮零点标准液浓度"=w266:dbl, "硝氮跨度标准液浓度"=w265:dbl, "硝氮标准液标准浓度"=w264:dbl)
        n190 = global read "总磷总氮断电保存全局变量.vi" "硝氮自动测试量程配置"() -> (w269:T10)
      }
      frame 6 {
        n191 = Unbundle By Name(w274) -> ("亚硝氮跨度值"=w273:dbl, "亚硝氮零点标准液浓度"=w272:dbl, "亚硝氮跨度标准液浓度"=w271:dbl, "亚硝氮标准液标准浓度"=w270:dbl)
        n192 = global read "总磷总氮断电保存全局变量.vi" "亚硝氮自动测试量程配置"() -> (w275:T10)
      }
      frame 7 {
        n193 = Unbundle By Name(w280) -> ("硅酸盐跨度值"=w279:dbl, "硅酸盐零点标准液浓度"=w278:dbl, "硅酸盐跨度标准液浓度"=w277:dbl, "硅酸盐标准液标准浓度"=w276:dbl)
        n194 = global read "总磷总氮断电保存全局变量.vi" "硅酸盐自动测试量程配置"() -> (w281:T10)
      }
      frame 8 {
        n195 = Unbundle By Name(w286) -> ("硫化物跨度值"=w285:dbl, "硫化物零点标准液浓度"=w284:dbl, "硫化物跨度标准液浓度"=w283:dbl, "硫化物标准液标准浓度"=w282:dbl)
        n196 = global read "总磷总氮断电保存全局变量.vi" "硫化物自动测试量程配置"() -> (w287:T10)
      }
      frame 22 {
        n197 = Unbundle By Name(w292) -> ("COD跨度值"=w291:dbl, "COD零点标准液浓度"=w290:dbl, "COD跨度标准液浓度"=w289:dbl, "COD标准液标准浓度"=w288:dbl)
        n198 = global read "总磷总氮断电保存全局变量.vi" "COD自动测试量程配置"() -> (w294:T10)
        n199 = global read "总磷总氮断电保存全局变量.vi" "CODcr消解时长"() -> (w293:dbl)
      }
    }
    "消解时长" <- w224
    n200 = global read "总磷总氮断电保存全局变量.vi" "IP"() -> (w233:string)
    n201 = local write "IP"(w233) -> ()
    n202 = Wait (ms)(milliseconds to wait=u32 1000 ("等待时间（毫秒）")) -> ()  [unwired: 1 out]
    n203 = local write "跨度值"(w226) -> ()
    n204 = local write "零点核查标液浓度"(w227) -> ()
    n205 = local write "跨度核查标液浓度"(w228) -> ()
    n206 = local write "标样核查标液浓度"(w229) -> ()
    n207 = To Unsigned Word Integer(number=w223) -> (unsigned 16bit integer=w222:T11)
    n208 = Unbundle By Name(w222) -> ("水样测试量程模式"=w221:u16, "空白核查量程模式"=w219:u16, "跨度核查量程模式"=w218:u16, "加标回收量程模式"=w217:u16, "标样核查量程模式"=w220:u16)
    n209 = local write "水样测试量程模式"(w221) -> ()
    n210 = local write "零点核查量程模式"(w219) -> ()
    n211 = local write "跨度核查量程模式"(w218) -> ()
    n212 = local write "加标回收量程模式"(w217) -> ()
    n213 = local write "标样核查量程模式"(w220) -> ()
  }
  n214 = while {
    tunnel: w2 -> [w305]
    tunnel: w3 -> [w304]
    tunnel: w4 -> [w303]
    tunnel: w1 -> [w302]
    stop <- FALSE stop-if-true
    n215 = Wait on Occurrence(2:w302) -> (0:w296:bool)  [unwired: 2 in]
    n216 = flat-sequence {
      tunnel: w305 -> [w312]
      tunnel: w304 -> [w311]
      tunnel: w303 -> [w310]
      tunnel: [w309] -> w299
      tunnel: [w308] -> w298
      tunnel: [w307] -> w297
      tunnel: w296 -> [_]
      frame #0 {
        n217 = property class="Enum (严格)"(reference=w310) -> ("Value"=w307:T1)  [unwired: 1 in, 2 out]
        n218 = property class="Enum (严格)"(reference=w311) -> ("Value"=w308:enum16{"低量程", "高量程"})  [unwired: 1 in, 2 out]
        n219 = property class="Ring (严格)"(reference=w312) -> ("Value"=w309:u16)  [unwired: 1 in, 2 out]
      }
    }
    n220 = flat-sequence {
      tunnel: [w315] -> w301
      tunnel: [w314] -> w300
      tunnel: w299 -> [w313]
      tunnel: w298 -> [w315]
      tunnel: w297 -> [w314]
      tunnel: [w313] -> w295
      tunnel: w301 -> [w334]
      tunnel: w300 -> [w335]
      tunnel: w295 -> [w333]
      frame #0 {
      }
      frame #1 {
        n221 = call "总磷总氮量程读取.vi"("测量参数"=w333) -> ("error out"=w324:errorcluster, "量程参数读取"=w332:T5)  [unwired: 9 in]
        n222 = Unbundle By Name(w332) -> ("测量精度"=→"测量精度":u16, "检出限"=→"检出限":dbl, "上限"=→"量程上限":dbl, "下限"=→"量程下限":dbl, "阈值（低->高）"=→"阈值（低->高）":dbl, "阈值（高->低）"=→"阈值（高->低）":dbl, "稀释度"=→"稀释度":dbl)
        n223 = call "总磷总氮公式读取.vi"("error in (no error)"=w324, "量程"=w334, "测量模式"=w335, "测量参数"=w333) -> ("error out"=w318:errorcluster, "公式"=w323:cluster{"X^2":dbl, "X":dbl, "b":dbl})  [unwired: 6 in]
        n224 = Unbundle By Name(w323) -> ("X^2"=→"二次多项式系数":dbl, "X"=→"曲线斜率":dbl, "b"=→"曲线截距":dbl)
        n225 = global read "VAR总磷总氮全局变量.vi" "MB session in"() -> (w317:refnum<class "MB_Master.lvclass">)
        n226 = case shown="1, 2, 22" w333 {
          tunnel: [_ w343] -> w319
          tunnel: [w336 w339] -> _
          tunnel: w318 -> [w336 w342]
          tunnel: w317 -> [_ w341]
          tunnel: [_ w337] -> w316
          frame 0, Default {
          }
          frame 1, 2, 22 {
            n227 = call "读取外设配置.vi"("error in (no error)"=w342, "MB session in"=w341) -> ("error out"=w340:errorcluster, "外设配置"=w344:T6, "MB session out"=w338:refnum<class "MB_Master.lvclass">)  [unwired: 7 in]
            n228 = Unbundle By Name(w344) -> ("消解温度下限"=w343:sgl)
            n229 = call "盐度补偿值读取.vi"("Error in"=w340, "MB session in"=w338) -> ("error out"=w339:errorcluster, "盐度补偿值"=w337:sgl)  [unwired: 7 in, 1 out]
          }
        }
        "消解温度" <- w319
        "盐度补偿值" <- w316
      }
      frame #2 {
        n230 = Format Date/Time String() -> (date/time string=→"数据刷新时间":string)  [unwired: 3 in]
      }
    }
  }
